vi "Write Winner_.vi"(8 "error in (no error)":errorcluster, 10 "Winner?":bool, 11 "SnakeGame in":refnum<class "SnakeGame.lvclass">) -> (0 "error out":errorcluster, 3 "SnakeGame out":refnum<class "SnakeGame.lvclass">)   [LabVIEW 2019, in "RT_Game.lvlib" / "SnakeGame.lvclass"]
uses:
  SnakeGame.lvclass
  SnakeGame.lvclass/SnakeGame.ctl
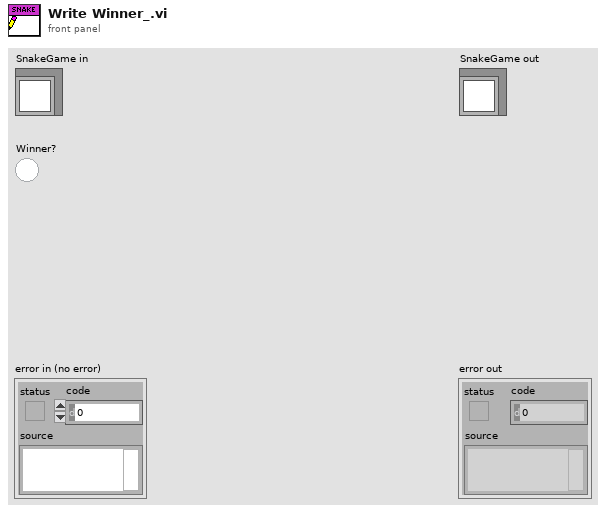
[diagram p1: front panel]
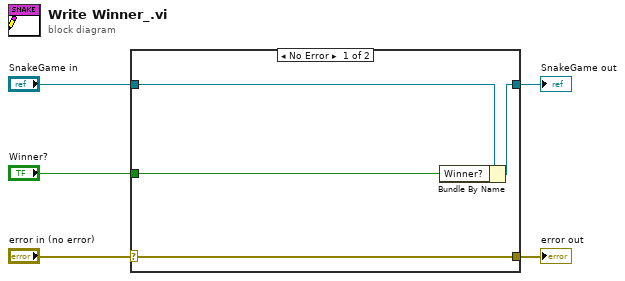
[diagram p0: block diagram]
diagram:
  n1 = case shown="No Error" "error in (no error)" {
    selector: "error in (no error)" -> [w9 w10]
    tunnel: [w9 w10] -> w4
    tunnel: [w7 w11] -> w2
    tunnel: "SnakeGame in" -> [w8 w11]
    tunnel: "Winner?" -> [w6 _]
    frame No Error {
      n2 = Bundle By Name(cluster=w8, "Winner?"=w6) -> (w7:refnum<class "SnakeGame.lvclass">)
    }
    frame Error {
    }
  }
  "error out" <- w4
  "SnakeGame out" <- w2
